vi "send on connection.vi"(8 "error in":errorcluster, 9 "timeout ms (10000)":i32=10000, 10 "data message":refnum<class "communicator message.lvclass">, 11 "connection in":refnum<class "TCP connection.lvclass">) -> (0 "error out":errorcluster, 3 "connection out":refnum<class "TCP connection.lvclass">)   [LabVIEW 2015, in "TCP connection.lvclass"]
uses:
  TCP connection.lvclass
  message/communicator message.lvclass
  TCP connection.lvclass/TCP connection.ctl
  TCP/TCP server.lvclass
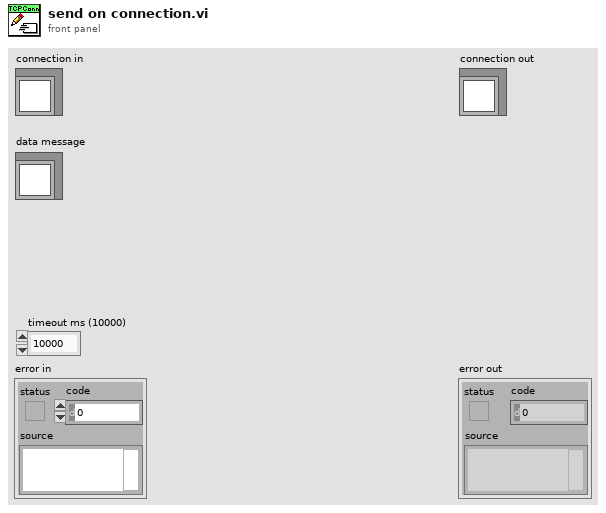
[diagram p1: front panel]
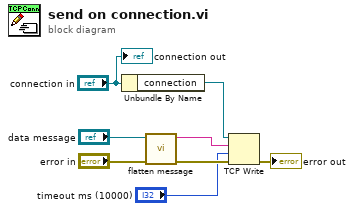
[diagram p0: block diagram]
diagram:
  n1 = Unbundle By Name("connection in") -> ("connection"=w6:refnum<k5>)
  n2 = call "flatten message.vi"("error in"="error in", "data message"="data message") -> ("error out"=w4:errorcluster, "data"=w5:string)  [unwired: 8 in]
  n3 = TCP Write(connection ID=w6, data in=w5, error in (no error)=w4, 9:"timeout ms (10000)") -> (error out=→"error out":errorcluster)  [unwired: 2 out]
  "connection out" <- "connection in"
